vi "Is slot valid.vi"(8 "error in (no error)":errorcluster, 10 "Card Position":T2={"Rack #"=0, "Slot #"=1} {"Slot #" max=15}, 11 "Device Ref in":T1 format="%.0x") -> (0 "error out":errorcluster, 2 "Valid?":bool, 3 "Device Ref out":T1 format="%.0x")   [LabVIEW 2014, in "SLSC configuration System Explorer.lvlib"]
uses:
  SLSC configuration System Explorer.lvlib
  <vilib>/NI Veristand/Custom Device API/Custom Device Item Ref.ctl
  Type Defs/Card Position.ctl
  Shared/SPI Utility/Slot #.ctl
  Shared/Constants.vi
  <vilib>/NI Veristand/Custom Device API/Get Item Property (U16).vi
  Shared/SLSC configuration Shared.lvlib
  <vilib>/NI Veristand/Custom Device API/Custom Device API.lvlib
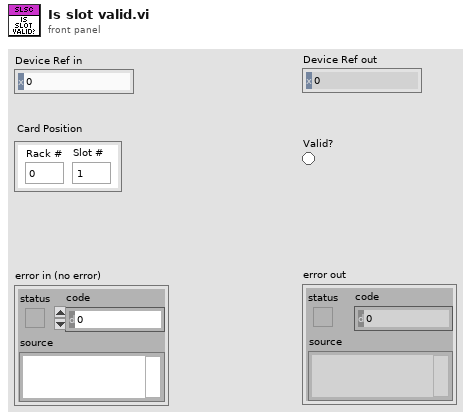
[diagram p1: front panel]
types:
  T1 = typedef "Custom Device API.lvlib/Custom Device Item Ref.ctl" = u64
  T2 = typedef "SLSC configuration Shared.lvlib/Card Position.ctl" = cluster{"Rack #":u8, "Slot #":T3}
  T3 = typedef "SLSC configuration Shared.lvlib/Slot #.ctl" = u8
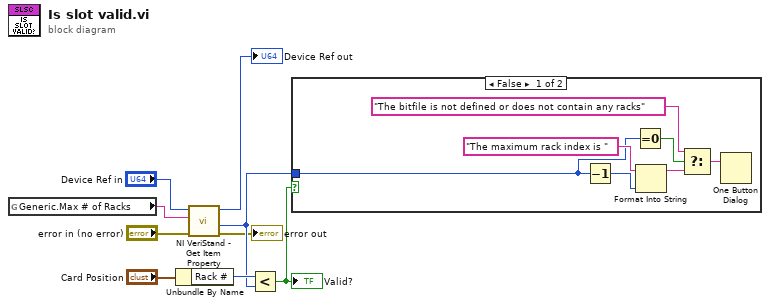
[diagram p0: block diagram]
diagram:
  n1 = global read "Constants.vi" "Generic.Max # of Racks"() -> (w8:string)
  n2 = Unbundle By Name("Card Position") -> ("Rack #"=w5:u8)
  n3 = call-poly <vilib>:"NI VeriStand - Get Item Property.vi"("error in (no error)"="error in (no error)", "Property Name"=w8, "Item Ref in"="Device Ref in") -> ("error out"=→"error out":errorcluster, "Value"=w4:u16, "Item Ref out"=→"Device Ref out":T1)  [unwired: 5 in, 1 out]
  n4 = Less?(x=w5, y=w4) -> (x < y?=w3:bool)
  "Valid?" <- w3
  n5 = case shown="False" w3 {
    tunnel: w4 -> [w10 _]
    frame False {
      n6 = Decrement(x=w10) -> (x-1=w12:u16)
      n7 = Equal To 0?(x=w10) -> (x = 0?=w13:bool)
      n8 = Format Into String(initial string="The maximum rack index is " ("message"), w12) -> (resulting string=w15:string)  [unwired: 2 in, 1 out]
      n9 = Select(t="The bitfile is not defined or does not contain any racks" ("message"), s=w13, f=w15) -> (s? t:f=w16:string)
      n10 = One Button Dialog(message=w16) -> ()  [unwired: 1 in, 1 out]
    }
    frame True {
    }
  }
